vi "Phasor Compute Standard Deviation (Poisson).vi"(0 "Time-Gated Decay":cluster{"t Array":dbl[], "I Array":dbl[]}, 5 "Phasor SDV Options in":T1, 9 "Phasor Frequency":dbl[unit], 11 "Error In":errorcluster, 12 "Calibration Phasor (m, phi)":T3={"m"=1.0, "phi"=0.0, "Phasor Frequency"=0.0, "Reference Lifetime"=0.0}, 13 "seed":i32=-1) -> (1 "(Mean) Phasor (g, s)":T2, 3 "Phasor SDV (g, s)":T2, 4 "Time-Gated Decay (dup)":cluster{"t Array":dbl[], "I Array":dbl[]}, 6 "Phasor SDV Options out":T1, 10 "Calibrated Phasor SDV (g, s)":T2, 14 "Calibrated (Mean) Phasor (g, s)":T2, 15 "Error Out":errorcluster)   [LabVIEW 2021, in "Phasor.lvlib"]
uses:
  Phasor.lvlib
  Phasor (g, s).ctl
  Phasor Standard Deviation Options.ctl
  Calibration Phasor (m, phi).ctl
  Phasor (m, phi).ctl
  250b1729-96e1-4389-8a25-986bf6130f6e.vi
  250b1729-96e1-4389-8a25-986bf6130f6e.vi/8a80743f-1319-44c8-96b0-3ef8fc688731.vi
  250b1729-96e1-4389-8a25-986bf6130f6e.vi/931f4f8f-d8c6-4056-833f-5c8fe97b24b9.vi
  <vilib>/Utility/error.llb/Error Cluster From Error Code.vi
  <vilib>/ErrorRing/Error Ring.xnode
  Error/Error.lvlib
  <vilib>/Analysis/NI_AALBase.lvlib
  Time/Time.lvlib
  Math/Math.lvlib
panel:
  out "CPU (s)":dbl
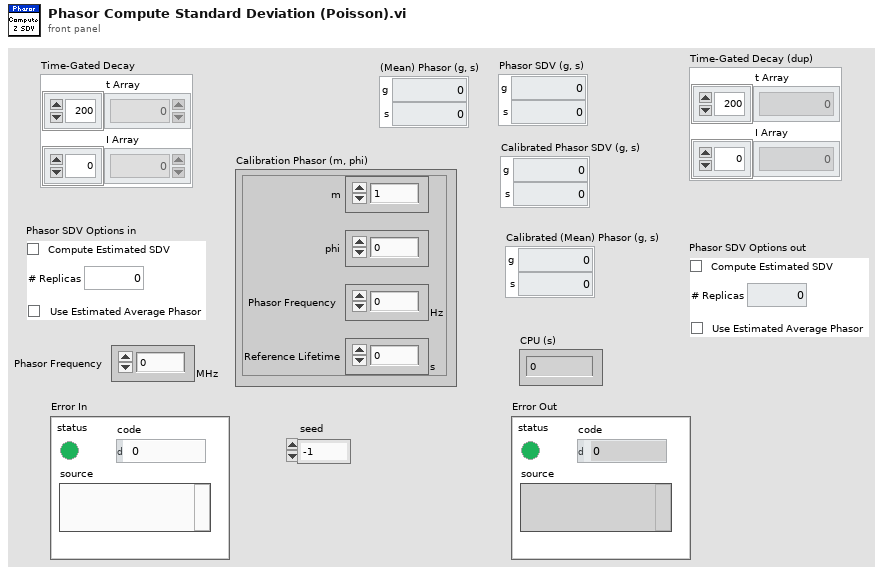
[diagram p1: front panel]
types:
  T1 = typedef "Phasor.lvlib/Phasor Standard Deviation Options.ctl" = cluster{"Compute Estimated SDV":bool, "# Replicas":u32, "Use Estimated Average Phasor":bool}
  T2 = typedef "Phasor.lvlib/Phasor (g, s).ctl" = cluster{"g":dbl, "s":dbl}
  T3 = typedef "Phasor.lvlib/Calibration Phasor (m, phi).ctl" = cluster{"m":dbl, "phi":dbl, "Phasor Frequency":dbl[unit], "Reference Lifetime":dbl[unit]}
  T4 = typedef "Phasor.lvlib/Phasor (m, phi).ctl" = cluster{"m":dbl, "phi":dbl}
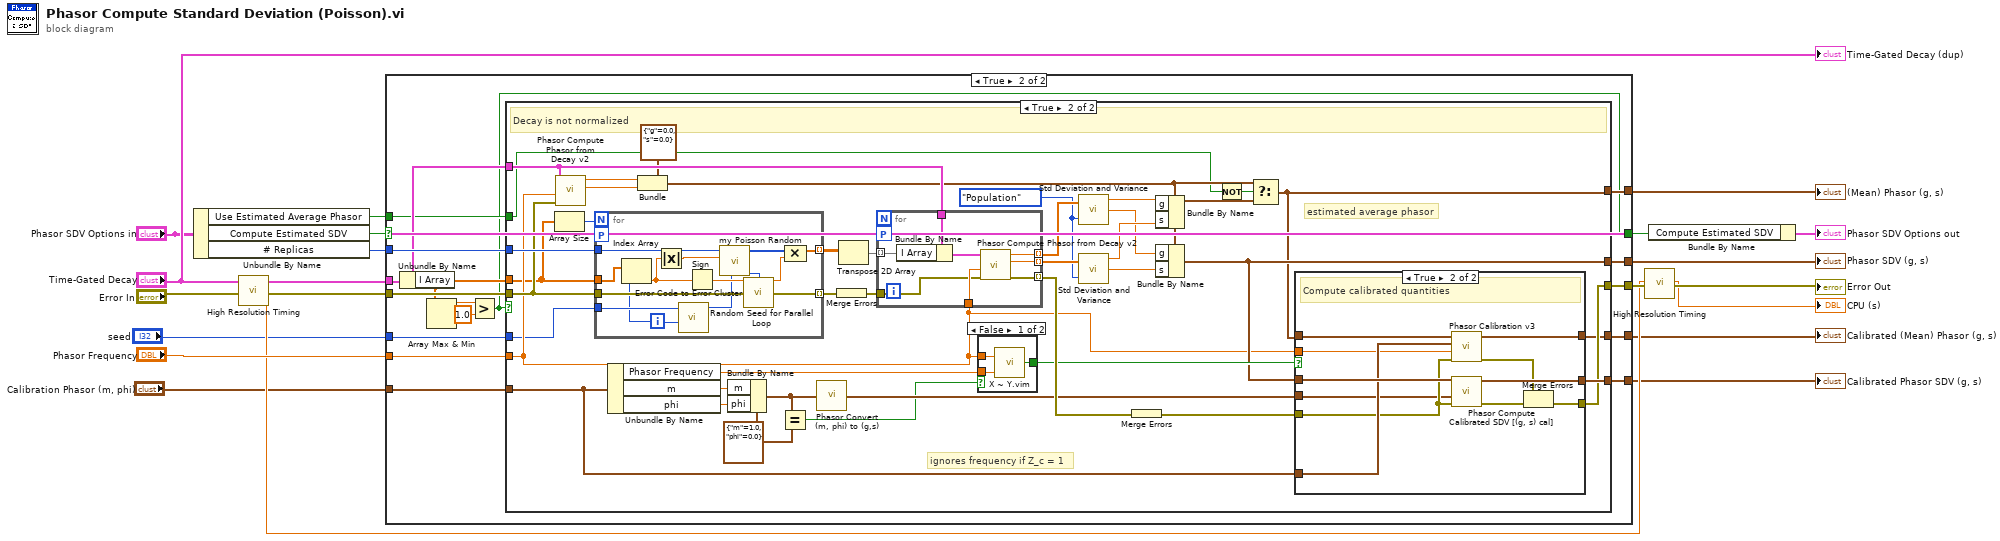
[diagram p0: block diagram]
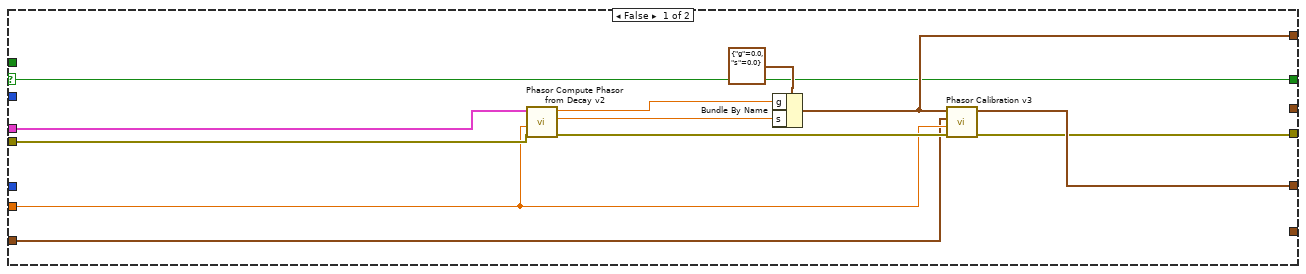
[diagram p2: hidden frame]
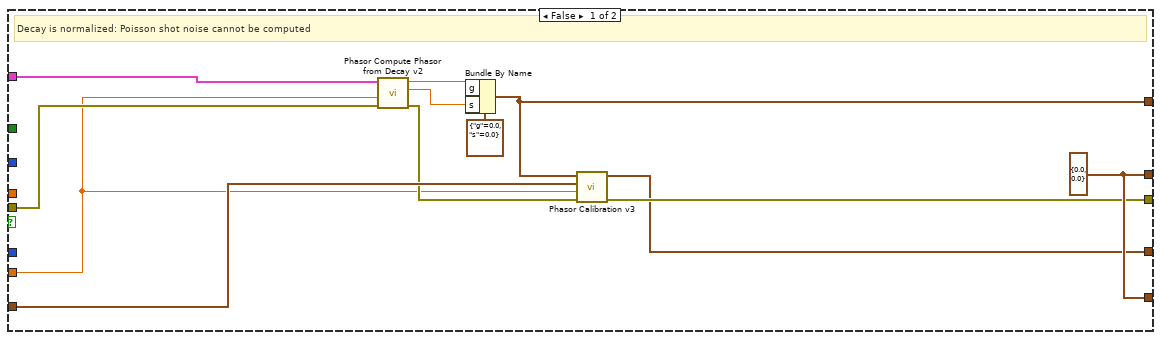
[diagram p3: hidden frame]
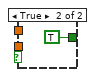
[diagram p4: hidden frame]
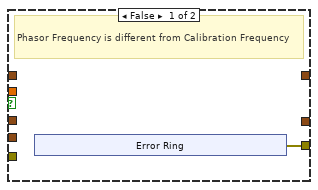
[diagram p5: hidden frame]
diagram:
  n1 = Unbundle By Name("Phasor SDV Options in") -> ("Use Estimated Average Phasor"=w5:bool, "Compute Estimated SDV"=w20:bool, "# Replicas"=w17:u32)
  n2 = call "High Resolution Timing.vi"("Error In"="Error In") -> ("elapsed (relative) seconds"=w11:dbl, "Error Out"=w13:errorcluster)  [unwired: 16 in, 1 out]
  n3 = case shown="True" w20 {
    selector: w20 -> [w21 _]
    tunnel: [_ w41] -> w19
    tunnel: "Time-Gated Decay" -> [w32 w44]
    tunnel: w17 -> [_ w48]
    tunnel: [w24 w40] -> w16
    tunnel: w13 -> [w31 w47]
    tunnel: "Phasor Frequency" -> [w23 w42]
    tunnel: [w27 w45] -> w9
    tunnel: "Calibration Phasor (m, phi)" -> [w22 w46]
    tunnel: [_ w43] -> w7
    tunnel: [w26 w36] -> w6
    tunnel: w5 -> [_ w35]
    tunnel: [w21 w34] -> w4
    tunnel: "seed" -> [_ w33]
    frame False {
      n4 = call "Phasor Compute Phasor from Decay v2.vi"("Error In"=w31, "Phasor Frequency"=w23, "Time-Gated Decay"=w32) -> ("Error Out"=w25:errorcluster, "s"=w28:dbl, "g"=w29:dbl)  [unwired: 5 in, 1 out]
      n5 = Bundle By Name(cluster=T2 {"g"=0.0, "s"=0.0} ("Phasor"), "g"=w29, "s"=w28) -> (w27:T2)
      n6 = call "Phasor Calibration v3.vi"("Error In"=w25, "Phasor Frequency"=w23, "Calibration Phasor"=w22, "Measured Phasor"=w27) -> ("Error Out"=w24:errorcluster, "Calibrated Phasor"=w26:T2)  [unwired: 2 in, 4 out]
    }
    frame True {
      n7 = Unbundle By Name(w44) -> ("I Array"=w39:dbl[])
      n8 = Array Max & Min(array=w39) -> (max value=w38:dbl)  [unwired: 3 out]
      n9 = Greater?(x=w38, y=1.0) -> (0:w34:bool)
      n10 = case shown="True" w34 {
        tunnel: w48 -> [_ w100]
        tunnel: w47 -> [w51 w72]
        tunnel: w46 -> [w54 w75]
        tunnel: [w53 w68] -> w45
        tunnel: w44 -> [w59 w73]
        tunnel: [w55 w92] -> w43
        tunnel: w42 -> [w50 w67]
        tunnel: [w55 w81] -> w41
        tunnel: [w52 w79] -> w40
        tunnel: w39 -> [_ w62]
        tunnel: [w49 w74] -> w36
        tunnel: w35 -> [_ w60]
        tunnel: w33 -> [_ w63]
        frame False {
          w55 = T2 {"g"=0.0, "s"=0.0} ("Phasor")
          # "Decay is normalized: Poisson shot noise cannot be computed"
          n11 = call "Phasor Compute Phasor from Decay v2.vi"("Error In"=w51, "Phasor Frequency"=w50, "Time-Gated Decay"=w59) -> ("Error Out"=w52:errorcluster, "s"=w56:dbl, "g"=w57:dbl)  [unwired: 5 in, 1 out]
          n12 = Bundle By Name(cluster=T2 {"g"=0.0, "s"=0.0} ("Phasor"), "g"=w57, "s"=w56) -> (w53:T2)
          n13 = call "Phasor Calibration v3.vi"("Error In"=w52, "Phasor Frequency"=w50, "Calibration Phasor"=w54, "Measured Phasor"=w53) -> ("Calibrated Phasor"=w49:T2)  [unwired: 2 in, 5 out]
        }
        frame True {
          w77 = T4 {"m"=1.0, "phi"=0.0} ("Phasor (m, phi)")
          w90 = enum16{"Sample", "Population"}."Population" ("Weighting (Sample)")
          # "estimated average phasor"
          # "ignores frequency if Z_c = 1"
          # "Decay is not normalized"
          n14 = Array Size(array=w62) -> (size(s)=w61:i32)
          n15 = call "Phasor Compute Phasor from Decay v2.vi"("Error In"=w72, "Phasor Frequency"=w67, "Time-Gated Decay"=w73) -> ("s"=w69:dbl, "g"=w70:dbl)  [unwired: 5 in, 2 out]
          n16 = for {
            N: w61 -> [_]
            tunnel: w62 -> [w136]
            tunnel: w100 -> [w141]
            workers-P: _ -> [_]
            tunnel: [w140] -> w99 mode=indexing
            tunnel: [w137] -> w98 mode=indexing
            tunnel: w72 -> [w139]
            tunnel: w63 -> [w132]
            i -> [w130]
            n17 = Index Array(array=w136, index=w130) -> (element=w131:dbl)
            n18 = Absolute Value(x=w131) -> (abs(x)=w138:dbl)
            n19 = call "Random Seed for Parallel Loop.vi"("Iteration"=w130, "Seed in (-1)"=w132) -> ("Seed out"=w129:i32)  [unwired: 9 in]
            n20 = Sign(1:w131) -> (0:w133:dbl)
            n21 = call "my Poisson Random.vi"("seed (-1)"=w129, "lambda"=w138, "samples (1)"=w141) -> ("error"=w134:i32, "Poisson random data"=w135:i32[])  [unwired: 7 in]
            n22 = call "Error Code to Error Cluster.vi"("Error Code"=w134, "Error In"=w139) -> ("Error Out"=w140:errorcluster)  [unwired: 13 in]
            n23 = Compound Arithmetic op=MULTIPLY(w135, w133) -> (w137:dbl[])
          }
          n24 = Unbundle By Name(w75) -> ("Phasor Frequency"=w91:dbl[unit], "m"=w84:dbl, "phi"=w83:dbl)
          n25 = Bundle(cluster=T2 {"g"=0.0, "s"=0.0} ("Phasor"), "g"=w70, "s"=w69) -> (w65:T2)
          n26 = Bundle By Name(cluster=w77, "m"=w84, "phi"=w83) -> (w78:T4)
          n27 = Equal?(x=w78, y=w77) -> (x = y?=w76:bool)
          n28 = call "Phasor Convert (m, phi) to (g,s).vi"("Phasor (m, phi)"=w78) -> ("Phasor (g, s)"=w82:T2)  [unwired: 8 in]
          n29 = Merge Errors(w99) -> (w96:errorcluster)
          n30 = Transpose 2D Array(2D array=w98) -> (transposed array=w97:dbl[][])
          n31 = for {
            tunnel: w97 -> [w128] mode=indexing
            tunnel: w73 -> [w127]
            tunnel: w67 -> [w126]
            tunnel: w96 -> [w125]
            workers-P: _ -> [_]
            tunnel: [w124] -> w94 mode=indexing
            tunnel: [w123] -> w93 mode=indexing
            tunnel: [w122] -> w95 mode=indexing
            n32 = Bundle By Name(cluster=w127, "I Array"=w128) -> (w121:cluster{"t Array":dbl[], "I Array":dbl[]})
            n33 = call "Phasor Compute Phasor from Decay v2.vi"("Error In"=w125, "Phasor Frequency"=w126, "Time-Gated Decay"=w121) -> ("Error Out"=w122:errorcluster, "s"=w123:dbl, "g"=w124:dbl)  [unwired: 5 in, 1 out]
          }
          n34 = case shown="False" w76 {
            tunnel: w91 -> [w103 _]
            tunnel: w67 -> [w102 _]
            tunnel: [w101 TRUE ("X ~= Y?")] -> w85
            frame False {
              n35 = call "X ~ Y.vim"("X"=w102, "Y"=w103) -> ("X ~= Y?"=w101:bool)  [unwired: 13 in]
            }
            frame True {
            }
          }
          n36 = call <vilib>:"Std Deviation and Variance.vi"("X"=w94, "Weighting (Sample)"=w90) -> ("mean"=w89:dbl, "standard deviation"=w87:dbl)  [unwired: 1 out]
          n37 = call <vilib>:"Std Deviation and Variance.vi"("X"=w93, "Weighting (Sample)"=w90) -> ("mean"=w88:dbl, "standard deviation"=w86:dbl)  [unwired: 1 out]
          n38 = Merge Errors(w95) -> (w80:errorcluster)
          n39 = Bundle By Name(cluster=w65, "g"=w89, "s"=w88) -> (w66:T2)
          n40 = Bundle By Name(cluster=w65, "g"=w87, "s"=w86) -> (w81:T2)
          n41 = Not(x=w60) -> (.not. x?=w64:bool)
          n42 = Select(t=w65, s=w64, f=w66) -> (s? t:f=w68:T2)
          n43 = case shown="True" w85 {
            tunnel: [_ w120] -> w92
            tunnel: w82 -> [_ w111]
            tunnel: w81 -> [_ w119]
            tunnel: w80 -> [_ w113]
            tunnel: [w105 w115] -> w79
            tunnel: w75 -> [_ w117]
            tunnel: [_ w116] -> w74
            tunnel: w67 -> [_ w114]
            tunnel: w68 -> [_ w110]
            frame False {
              # "Phasor Frequency is different from Calibration Frequency"
              n44 = xnode "Error Ring"() -> ("error out"=w105:errorcluster)
            }
            frame True {
              # "Compute calibrated quantities"
              n45 = call "Phasor Calibration v3.vi"("Error In"=w113, "Phasor Frequency"=w114, "Calibration Phasor"=w117, "Measured Phasor"=w110) -> ("Error Out"=w112:errorcluster, "Calibrated Phasor"=w116:T2)  [unwired: 2 in, 4 out]
              n46 = call "Phasor Compute Calibrated SDV [(g, s) cal].vi"("Error In"=w113, "Phasor Calibration (g,s)"=w111, "Raw Phasor SDV (g, s)"=w119) -> ("Error Out"=w118:errorcluster, "Calibrated Phasor SDV (g, s)"=w120:T2)  [unwired: 7 in]
              n47 = Merge Errors(w112, w118) -> (w115:errorcluster)
            }
          }
        }
      }
    }
  }
  "Phasor SDV (g, s)" <- w19
  "(Mean) Phasor (g, s)" <- w9
  "Calibrated Phasor SDV (g, s)" <- w7
  "Calibrated (Mean) Phasor (g, s)" <- w6
  n48 = call "High Resolution Timing.vi"("relative seconds (NaN)"=w11, "Error In"=w16) -> ("elapsed (relative) seconds"=→"CPU (s)":dbl, "Error Out"=→"Error Out":errorcluster)  [unwired: 15 in, 1 out]
  n49 = Bundle By Name(cluster="Phasor SDV Options in", "Compute Estimated SDV"=w4) -> (→"Phasor SDV Options out":T1)
  "Time-Gated Decay (dup)" <- "Time-Gated Decay"
